vi "Auto_calibrate.vi"(3 "Mode":T4, 5 "Traverse line":T5 {"Row Duration (mins)" format="%#.1f"; "Row No" min=0; "Trace Gas Concentration (%)" min=0.0 format="%#.2f"; "Emission Rate (l/min)" format="%#.2f"; "Tunnel Speed" format="%#.2f"; "Start X" format="%#.2f"; "Start Y" format="%#.2f"; "Start Z" format="%#.2f"; "End X" format="%#.2f"; "End Y" format="%#.2f"; "End Z" format="%#.2f"; "Averaging time (min)" min=0.0 format="%#.2f"}) -> (0 "Error Messages":string, 1 "Status":T2, 2 "Traverse Out":T5 {"Row Duration (mins)" format="%#.1f"; "Row No" min=0; "Trace Gas Concentration (%)" min=0.0 format="%#.2f"; "Emission Rate (l/min)" format="%#.2f"; "Tunnel Speed" format="%#.2f"; "Start X" format="%#.2f"; "Start Y" format="%#.2f"; "Start Z" format="%#.2f"; "End X" format="%#.2f"; "End Y" format="%#.2f"; "End Z" format="%#.2f"; "Averaging time (min)" min=0.0 format="%#.2f"})   [LabVIEW 2010]
uses:
  Gen Trav/Traverse_cluster.ctl
  Gen Trav/Spacing.ctl
  Controls/Multi_run_mode.ctl
  Controls/User_Specific_mode.ctl
  Controls/Auto_Calib_Type.ctl
  Gen Trav/Multi_Run_Status.ctl
  Controls/Auto_Calib_Case.ctl
  File/Setup_Filetype.ctl
  Calibration/Calib_mode.ctl
  Controls/Save_Data.ctl
  Controls/Post_Process.ctl
  Controls/Setup.ctl
  Globals/Meas_global.vi
  Globals/Calib_global.vi
  Globals/Trav_pos_global.vi
  Globals/Plug_in_data_global.vi
  Globals/Extra_Commands_Global.vi
  <vilib>/Analysis/NI_AALBase.lvlib
panel:
  out "Minimum St Dev":dbl[](array[numeric])
  out "Time FFID valve moved":dbl
  out "Wait factor":dbl
  out "Establishment time":string
  out "Orig Calib file string":string
  out "Concentrations":dbl[](array[numeric])
  out "FFID St Dev":dbl[][](array[numeric]) format="%.2f"
  in  "Clear Calib History":bool
  out "Coefficients":dbl[][](array[numeric]) format="%.2f"
  out "Currently in Case":T1
  out "Valve position":dbl format="%.2f"
  out "Currently On":i32
  out "Values":dbl[][](array[numeric]) format="%.2f"
  out "FF Indexes":i16[](array[numeric])
  out "Ch No's":i16[](array[numeric])
  out "No of Calib Points":i32
  out "Root Name":string[](array[string])
  out "Original Calib File":path
  out "Calibration varying":T3
  in  "stop":bool
  out "New Calib Filenames":path[](array[path])
  # "Specific Argument Options\n      Tunnel Speed;1;2;3;4\nOR  Traverse Position\nOR   Concentration"
  # "X           Y            Z"
  # "Start"
  # "End"
  # "X           Y            Z"
  # "Start"
  # "End"
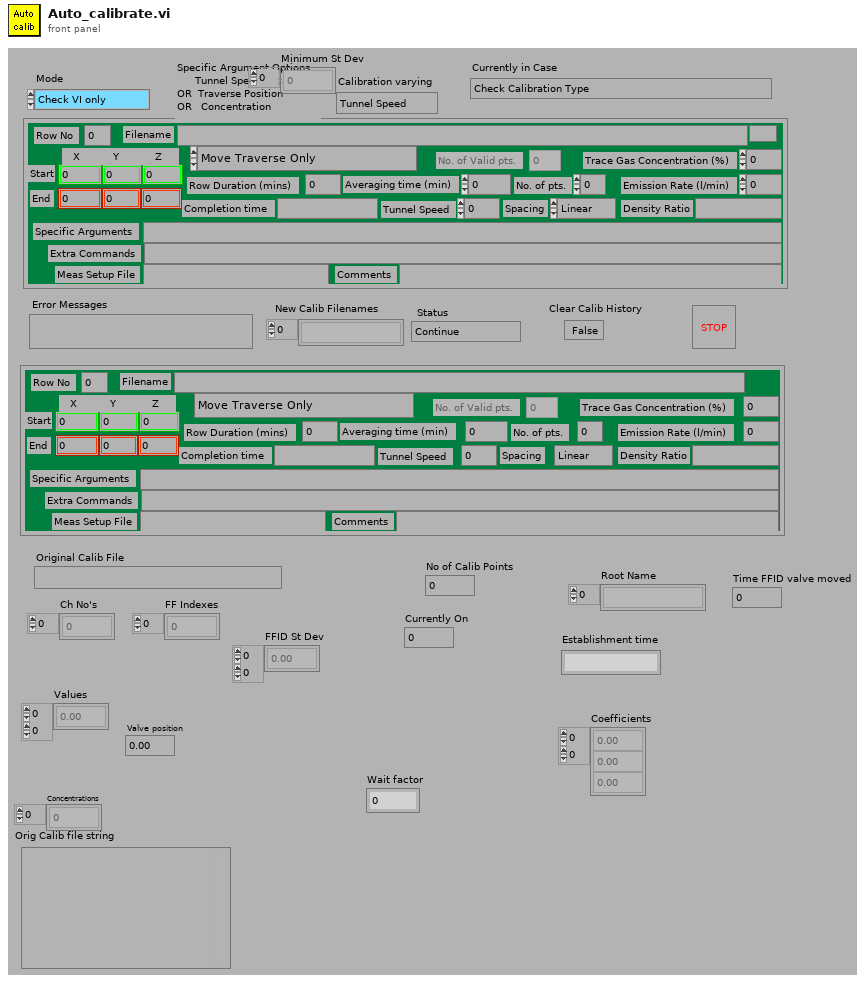
[diagram p1: front panel]
types:
  T1 = typedef "Auto_Calib_Case.ctl" = enum16{"Check Calibration Type", "Check if Original Calib file is Valid", "Get sampling rate etc. from meas setup file", "Setup Calibration Program", "Get Channel Numbers", "Check use latest selected on Mesurement setup files", "Create New Calib Filenames", "Setup Calibration Values in 2D array", "Create Measurement Setup File (Concentration Only)", "Are There Enough Calibration Points", "Set Measurement Conditions", "Measure Calibration Point", "Do Another Calibration Point?", "Skip Next Frame?", "Insert New calibration Filenames into Measurement Setup file", "Warn if FFID calibration is very non linear", "Warn if FFID variance is high", "Insert Bkgnd Variance into calib file", "Warn if FFID voltages are too low", "Warn if Current Calibration fit is poor", "Warn if Calibration Coefficients have significantly altered", "End"}
  T2 = typedef "Multi_Run_Status.ctl" = enum16{"Continue", "Jump to Next Point", "Jump to Next Row", "Jump To Fall Back", "Terminate Run"}
  T3 = typedef "Auto_Calib_Type.ctl" = enum16{"Tunnel Speed", "Traverse Position", "Concentration"}
  T4 = typedef "User_Specific_mode.ctl" = enum16{"Check VI only", "Run VI"}
  T5 = typedef "Traverse_cluster.ctl" = cluster{"Start X":dbl, "Start Y":dbl, "Start Z":dbl, "End X":dbl, "End Y":dbl, "End Z":dbl, "No. of pts.":i32, "Spacing":T6, "Filename":path, "Tunnel Speed":dbl, "Averaging time (min)":dbl, "Extra Commands":string, "Specific Arguments":string, "Emission Rate (l/min)":dbl, "Trace Gas Concentration (%)":dbl, "Density Ratio":string, "Comments":string, "Row No":i32, "Row Type Selector":T7, "Completion time":string, "Row Duration (mins)":dbl, "No. of Valid pts.":i32, "Meas Setup File":string}
  T6 = typedef "Spacing.ctl" = enum16{"Linear", "Log", "Gauss", "Specified", "N/A"}
  T7 = typedef "Multi_run_mode.ctl" = enum16{"Move Traverse Only", "Set Tunnel Speed Only", "Set Source Only", "Set Measurement Conditions", "Single Measurement", "Vertical Profile", "Lateral Profile", "Longitudinal Profile", "Explore Volume", "Multi-Axis Profile", "Auto Calibrate", "Meas Fast FID Bkgnd", "Check Beam Power", "Scanning Valve Measurement", "Run VI Named:", "Set ADAM Ch", "Wait (minutes)", "Send Message", "Synchronize With:", "Fall Back to this Row", "Turn Off Row Repeating", "Blank Row"}
  T8 = typedef "Setup_Filetype.ctl" = enum16{"Measurement Setups", "Calibration Setups", "General", "Results File Plotter Setups", "Speed Calib Tweaks"}
  T9 = typedef "Calib_mode.ctl" = enum16{"Show Setup", "Take a New Calibration Point", "Refit Curve", "Setup Front Panel"}
  T10 = typedef "Save_Data.ctl" = enum16{"Save No Data", "Save Data"}
  T11 = typedef "Post_Process.ctl" = enum16{"Take New Data", "Post Process Raw Data File"}
  T12 = typedef "Setup.ctl" = enum16{"Run Program", "Show Setup", "Save Current Setup", "Setup Front Panel"}
  T13 = typedef "Cal_Inst_type.ctl" = enum16{"Propeller anemometer", "Pressure Transducer", "Hot wire", "Cross wire velocity", "Cross wire angle", "Generic Linear", "Generic Polynomial", "Generic BackPoly", "Fast FID", "Thermocouple", "Cold wire", "Pulsed Wire"}
  T14 = typedef "Ref_Inst_type.ctl" = enum16{"Propellor anemometer", "Pressure Transducer", "Raw voltage", "Pitot-static tube", "Preston tube", "Generic Linear", "Generic Polynomial", "Thermocouple", "LDA", "Enter Value", "ADAM Channel"}
  T15 = cluster{"2nd Ref type":T14, "2nd inst present":bool}
  T16 = cluster{"high limit (10V)":sgl, "low limit (-10V)":sgl, "Ch No":i16, "Var name":string}[]
  T17 = cluster{"high limit (10V)":sgl, "low limit (-10V)":sgl, "Ch No":i16, "Var name":string}
  T18 = typedef "Inst_type.ctl" = enum16{"Propeller anemometer", "Raw voltage", "Pressure Transducer", "Pitot-static tube", "Preston tube", "Hot wire", "Cross wire 1", "Cross wire 2", "Generic Linear", "Generic Polynomial", "Generic BackPoly", "Fast FID", "Thermocouple", "Cold wire", "Pulsed Wire", "LDA Vel", "LDA Tran time", "LDA Arr time"}
  T19 = cluster{"high limit (10V)":sgl, "low limit (-10V)":sgl, "Ch No":i16, "Calib filename":path, "Inst type":T18, "Symbol":string, "Move channel":bool, "Use Latest":bool, "D":dbl, "Ch Name":string}[]
  T20 = typedef "Status_Cluster.ctl" = cluster{"Status":T2, "Error Type":string, "Error Description":string}
  T21 = typedef "Valco_valve_ph.ctl" = u16
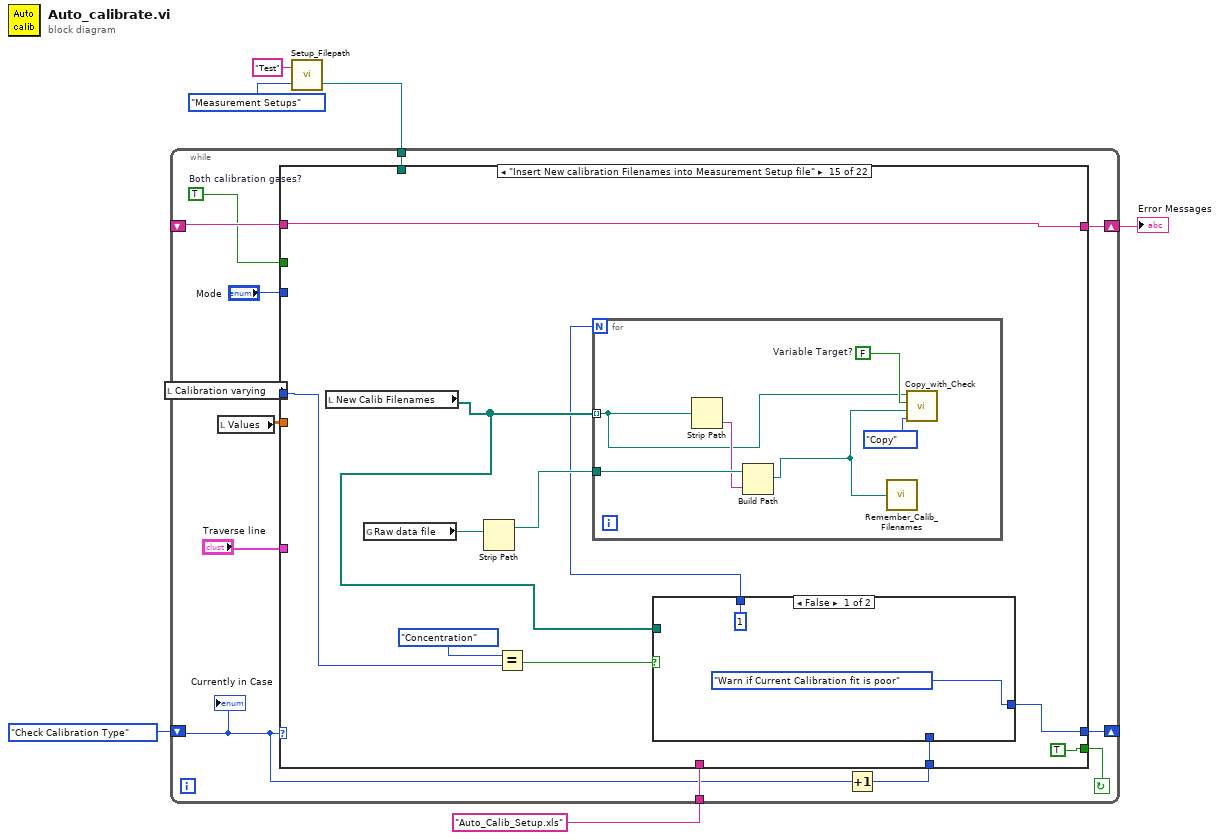
[diagram p0: block diagram]
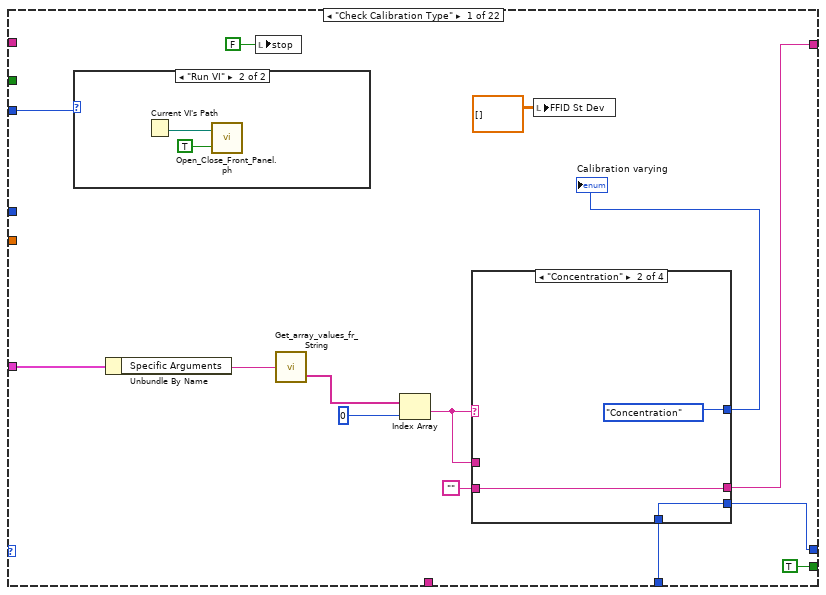
[diagram p2: hidden frame]
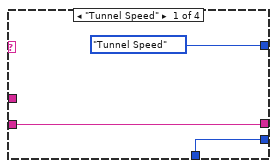
[diagram p4: hidden frame]
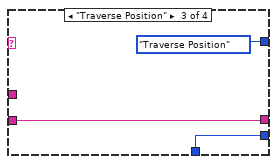
[diagram p5: hidden frame]
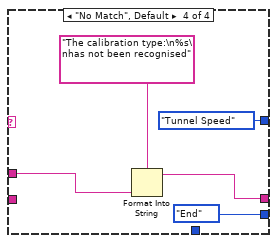
[diagram p6: hidden frame]
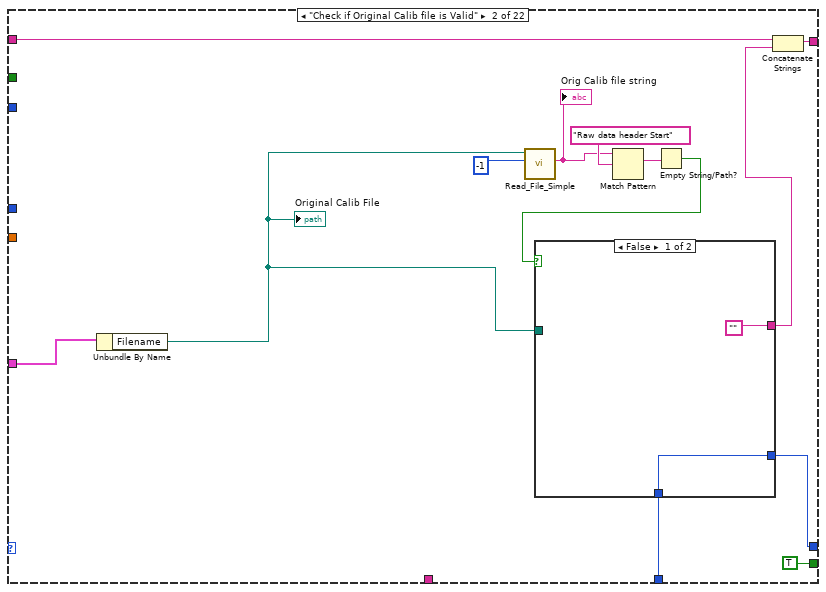
[diagram p7: hidden frame]
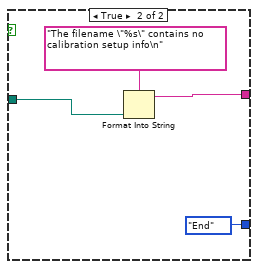
[diagram p8: hidden frame]
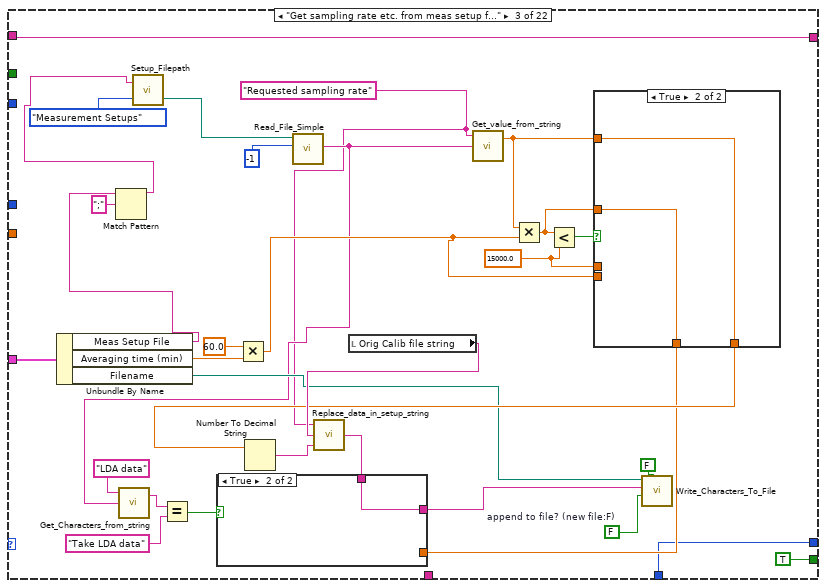
[diagram p9: hidden frame]
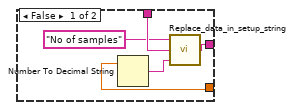
[diagram p10: hidden frame]
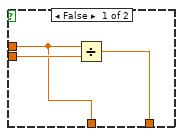
[diagram p11: hidden frame]
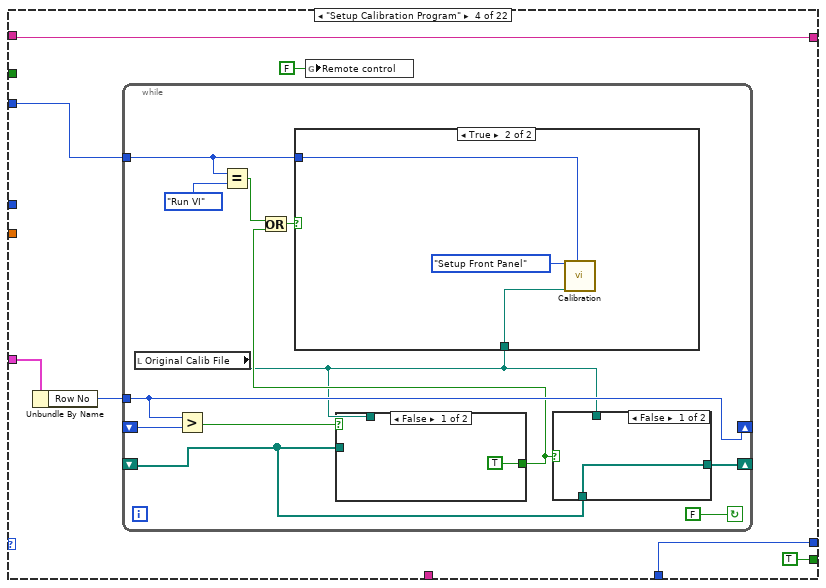
[diagram p12: hidden frame]
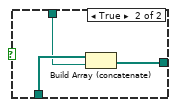
[diagram p13: hidden frame]
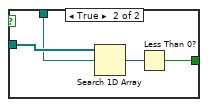
[diagram p15: hidden frame]
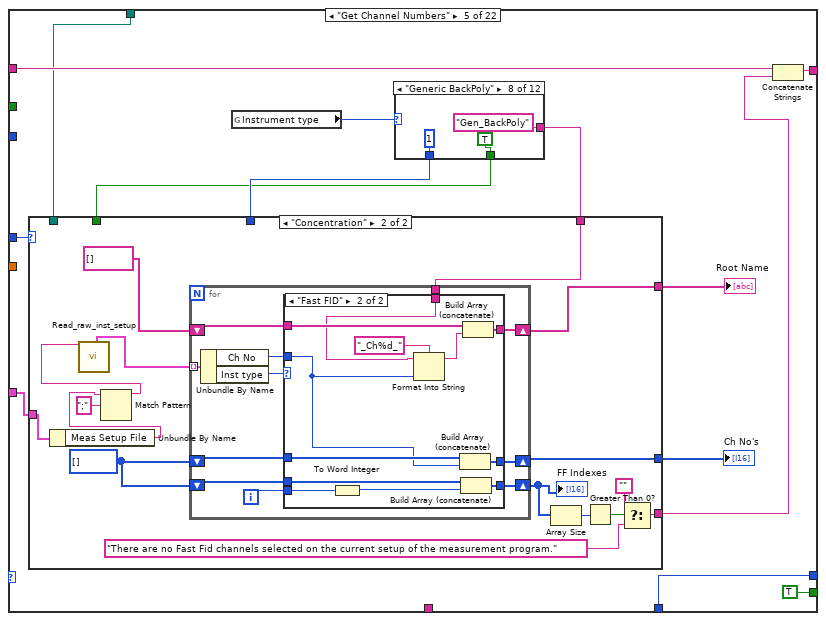
[diagram p16: hidden frame]
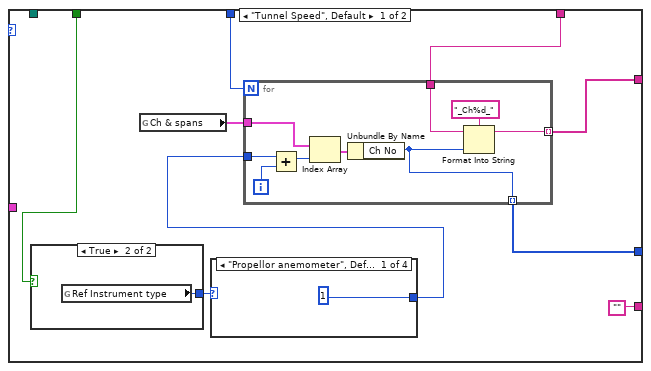
[diagram p17: hidden frame]
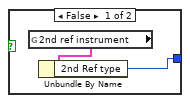
[diagram p18: hidden frame]
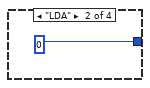
[diagram p19: hidden frame]
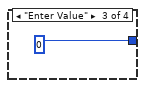
[diagram p20: hidden frame]
diagram:
  n1 = call "Setup_Filepath.vi"("Setup File Type"=Setup_Filetype."Measurement Setups", "Filename in"="Test") -> ("Filename Out"=w2:path)  [unwired: 1 out]
  n2 = while {
    shift-left: _ -> [w11]
    shift-right: [w12] -> w5
    shift-left: Auto_Calib_Case."Check Calibration Type" ("Currently in Case") -> [w10]
    shift-right: [w9] -> _
    tunnel: "Auto_Calib_Setup.xls" -> [w19]
    tunnel: w2 -> [w7]
    stop <- w15 continue-if-true
    w8 = TRUE  # Both calibration gases?
    n3 = local read "Calibration varying"() -> (w14:T3)
    n4 = local read "Values"() -> (w13:dbl[][])
    n5 = Increment(x=w10) -> (x+1=w16:T1)
    n6 = case shown="\"Insert New calibration Filenames into Measurement Setup file\"" w10 {
      tunnel: "Traverse line" -> [w33 w62 w100 w114 w145 _ _ w367 w400 _ w577 _ _ _ _ _ _ _ _ _ w991 w1022]
      tunnel: "Mode" -> [w24 _ _ w115 _ _ w318 _ w401 _ w572 _ w737 _ _ _ _ _ _ _ _ w1023]
      tunnel: w19 -> [_ _ _ _ _ _ _ _ w405 _ _ w649 _ _ _ _ _ _ _ _ _ _]
      tunnel: [w22 w52 w82 w117 w148 w264 w315 w358 w403 w540 w565 w648 w738 w764 w774 w793 w831 w896 w914 w970 w1014 w1028] -> w9
      tunnel: w16 -> [w23 w51 w82 w117 w148 w264 w315 w359 w403 w539 w559 w648 _ w763 w773 w793 w831 w896 w914 w970 w1014 w1028]
      tunnel: [TRUE TRUE TRUE TRUE TRUE TRUE TRUE TRUE w399 TRUE TRUE TRUE TRUE TRUE TRUE TRUE TRUE TRUE TRUE TRUE TRUE FALSE] -> w15
      tunnel: w14 -> [_ _ _ _ w152 _ w314 w365 _ _ w563 w650 w736 w762 w776 _ _ _ _ _ _ w1024]
      tunnel: w13 -> [_ _ _ _ _ _ _ _ w398 w549 w576 _ _ _ _ _ w838 _ w920 _ _ _]
      tunnel: [w26 w54 w80 w118 w149 w265 w329 w362 w404 w543 w560 w646 w735 w767 w780 w802 w845 w892 w921 w959 w1007 w1027] -> w12
      tunnel: w11 -> [_ w56 w80 w118 w151 w265 w329 w361 w404 w544 w560 w646 w735 w767 w780 w802 w845 w892 w921 w959 w1007 w1027]
      tunnel: w8 -> [_ _ _ _ _ _ _ w360 _ _ _ _ _ _ _ _ _ _ _ _ _ w1021]
      tunnel: w7 -> [_ _ _ _ w144 w267 _ _ w402 _ _ _ _ _ _ _ _ _ _ _ _ _]
      frame "Check Calibration Type" {
        n7 = case shown="\"Run VI\"" w24 {
          frame "Check VI only" {
          }
          frame "Run VI" {
            n8 = Current VI's Path() -> (path=w34:path)
            n9 = call "Open_Close_Front_Panel.ph.vi"("Front Panel Window:Open"=TRUE, "VI path"=w34) -> ()  [unwired: 2 out]
          }
        }
        n10 = Unbundle By Name(w33) -> ("Specific Arguments"=w32:string)
        n11 = local write "stop"(FALSE) -> ()
        n12 = call "Get_array_values_fr_String.vi"("String Value"=w32) -> ("String array"=w31:string[])  [unwired: 1 out]
        n13 = Index Array(array=w31, index=0 ("Index")) -> (element=w29:string)
        n14 = case shown="\"Concentration\"" w29 {
          tunnel: [Auto_Calib_Type."Tunnel Speed" ("Calibration varying") Auto_Calib_Type."Concentration" ("Calibration varying") Auto_Calib_Type."Traverse Position" ("Calibration varying") Auto_Calib_Type."Tunnel Speed" ("Calibration varying")] -> w27
          tunnel: w29 -> [_ _ _ w48]
          tunnel: [w37 w40 w43 w46] -> w26
          tunnel: "" -> [w37 w40 w43 _]
          tunnel: w23 -> [w36 w39 w42 _]
          tunnel: [w36 w39 w42 Auto_Calib_Case."End" ("Currently in Case")] -> w22
          frame "Tunnel Speed" {
          }
          frame "Concentration" {
            (unwired) ""
          }
          frame "Traverse Position" {
          }
          frame "No Match", Default {
            n15 = Format Into String(format string="The calibration type:\n%s\nhas not been recognised" ("Format String"), w48) -> (resulting string=w46:string)  [unwired: 2 in, 1 out]
          }
        }
        "Calibration varying" <- w27
        n16 = local write "FFID St Dev"(dbl[][] [] ("FFID Variance")) -> ()
      }
      frame "Check if Original Calib file is Valid" {
        n17 = Unbundle By Name(w62) -> ("Filename"=w50:path)
        "Original Calib File" <- w50
        n18 = call "Read_File_Simple.vi"("Filename"=w50, "number of characters (all:-1)"=-1) -> ("string"=w59:string)  [unwired: 1 in, 7 out]
        "Orig Calib file string" <- w59
        n19 = Match Pattern(string=w59, regular expression="Raw data header Start") -> (match substring=w58:string)  [unwired: 4 out]
        n20 = Empty String/Path?(string/path=w58) -> (empty?=w57:bool)
        n21 = case shown="False" w57 {
          tunnel: w50 -> [_ w68]
          tunnel: ["" w66] -> w55
          tunnel: [w63 Auto_Calib_Case."End" ("Currently in Case")] -> w52
          tunnel: w51 -> [w63 _]
          frame False {
          }
          frame True {
            n22 = Format Into String(format string="The filename \"%s\" contains no calibration setup info\n" ("Format String"), w68) -> (resulting string=w66:string)  [unwired: 2 in, 1 out]
          }
        }
        n23 = Concatenate Strings(w56, w55) -> (w54:string)
      }
      frame "Get sampling rate etc. from meas setup file" {
        w83 = FALSE  # append to file? (new file:F)
        w72 = "Requested sampling rate"
        w90 = 15000.0 ("y")
        n24 = Unbundle By Name(w100) -> ("Meas Setup File"=w78:string, "Averaging time (min)"=w98:dbl, "Filename"=w85:path)
        n25 = Match Pattern(string=w78, regular expression=";") -> (before substring=w70:string)  [unwired: 4 out]
        n26 = call "Setup_Filepath.vi"("Setup File Type"=Setup_Filetype."Measurement Setups", "Filename in"=w70) -> ("Filename Out"=w69:path)  [unwired: 1 out]
        n27 = Multiply(x=60.0, y=w98) -> (x*y=w89:dbl)
        n28 = call "Read_File_Simple.vi"("Filename"=w69, "number of characters (all:-1)"=-1) -> ("string"=w77:string)  [unwired: 1 in, 7 out]
        n29 = call "Get_Characters_from_string.vi"("Input string"=w77, "Variable name"="LDA data") -> ("Value"=w75:string)  [unwired: 1 in, 1 out]
        n30 = Equal?(x=w75, y="Take LDA data") -> (x = y?=w73:bool)
        n31 = local read "Orig Calib file string"() -> (w94:string)
        n32 = call "Get_value_from_string.vi"("Input string"=w77, "Variable name"=w72) -> ("Value"=w93:dbl)  [unwired: 1 in, 1 out]
        n33 = Multiply(x=w93, y=w89) -> (x*y=w88:dbl)
        n34 = Less?(x=w88, y=w90) -> (x < y?=w96:bool)
        n35 = case shown="True" w96 {
          tunnel: w93 -> [_ w111]
          tunnel: [w108 w111] -> w92
          tunnel: w90 -> [w107 _]
          tunnel: w89 -> [w109 _]
          tunnel: [w107 w110] -> w86
          tunnel: w88 -> [_ w110]
          frame False {
            n36 = Divide(x=w107, y=w109) -> (x/y=w108:dbl)
          }
          frame True {
          }
        }
        n37 = Number To Decimal String(number=w92) -> (decimal integer string=w91:string)  [unwired: 1 out]
        n38 = call "Replace_data_in_setup_string.vi"("New data string"=w91, "Input string"=w94, "Variable name"=w72) -> ("Appended string"=w87:string)
        n39 = case shown="True" w73 {
          tunnel: w87 -> [w105 w106]
          tunnel: w86 -> [w102 _]
          tunnel: [w101 w106] -> w84
          frame False {
            n40 = Number To Decimal String(number=w102) -> (decimal integer string=w103:string)  [unwired: 1 out]
            n41 = call "Replace_data_in_setup_string.vi"("New data string"=w103, "Input string"=w105, "Variable name"="No of samples") -> ("Appended string"=w101:string)
          }
          frame True {
          }
        }
        n42 = call "Write_Characters_To_File.vi"("file path (dialog if empty)"=w85, "advisory dialog? (display:T)"=FALSE, "character string"=w84, "append to file? (new file:F)"=w83) -> ()  [unwired: 1 in, 4 out]
      }
      frame "Setup Calibration Program" {
        n43 = Unbundle By Name(w114) -> ("Row No"=w113:i32)
        n44 = while {
          shift-left: _ -> [w122]
          shift-right: [w120] -> _
          tunnel: w113 -> [w129]
          shift-left: _ -> [w130]
          shift-right: [w129] -> _
          tunnel: w115 -> [w127]
          stop <- FALSE continue-if-true
          n45 = local read "Original Calib File"() -> (w121:path)
          n46 = Greater?(x=w129, y=w130) -> (0:w128:bool)
          n47 = Equal?(x=w127, y=User_Specific_mode."Run VI" ("Mode")) -> (x = y?=w125:bool)
          n48 = case shown="False" w128 {
            tunnel: w122 -> [_ w142]
            tunnel: w121 -> [_ w141]
            tunnel: [TRUE w139] -> w123
            frame False {
            }
            frame True {
              n49 = Search 1D Array(1D array=w142, element=w141) -> (index of element=w140:i32)  [unwired: 1 out]
              n50 = Less Than 0?(x=w140) -> (x < 0?=w139:bool)
            }
          }
          n51 = Or(x=w125, y=w123) -> (x .or. y?=w124:bool)
          n52 = case shown="True" w124 {
            tunnel: w127 -> [_ w137]
            tunnel: w121 -> [_ w136]
            frame False {
            }
            frame True {
              n53 = call "Calibration.vi"("Mode"=Calib_mode."Setup Front Panel", "Calib file"=w136, "Simulate/Run"=w137) -> ()  [unwired: 17 out]
            }
          }
          n54 = case shown="False" w123 {
            tunnel: w122 -> [w131 w134]
            tunnel: w121 -> [_ w133]
            tunnel: [w131 w132] -> w120
            frame False {
            }
            frame True {
              n55 = Build Array (concatenate)(w134, w133) -> (w132:path[])
            }
          }
        }
        n56 = global write "Meas_global.vi" "Remote control"(FALSE ("Remote control")) -> ()
      }
      frame "Get Channel Numbers" {
        n57 = global read "Calib_global.vi" "Instrument type"() -> (w156:T13)
        n58 = case shown="\"Generic BackPoly\"" w156 {
          tunnel: ["Prop" "Mano" "HW" "XW" "XW" "Gen_Lin" "Gen_Poly" "Gen_BackPoly" "FF" "Therm" "CW" "PWA"] -> w155
          tunnel: [1 1 1 2 2 1 1 1 1 1 1 1] -> w146
          tunnel: [TRUE TRUE TRUE TRUE FALSE TRUE TRUE TRUE TRUE TRUE TRUE TRUE] -> w143
          frame "Propeller anemometer" {
          }
          frame "Pressure Transducer" {
          }
          frame "Hot wire" {
          }
          frame "Cross wire velocity" {
          }
          frame "Cross wire angle" {
          }
          frame "Generic Linear" {
          }
          frame "Generic Polynomial" {
          }
          frame "Generic BackPoly" {
          }
          frame "Fast FID" {
          }
          frame "Thermocouple" {
          }
          frame "Cold wire" {
          }
          frame "Pulsed Wire" {
          }
        }
        n59 = case shown="\"Concentration\"" w152 {
          tunnel: w155 -> [w163 w197]
          tunnel: [w159 w196] -> w154
          tunnel: [w160 w194] -> w153
          tunnel: ["" w187] -> w150
          tunnel: w146 -> [w161 _]
          tunnel: w145 -> [_ w186]
          tunnel: w144 -> [_ _]
          tunnel: w143 -> [w157 _]
          frame "Tunnel Speed", Default {
            n60 = case shown="True" w157 {
              tunnel: [w166 w168] -> w165
              frame False {
                n61 = global read "Calib_global.vi" "2nd ref instrument"() -> (w167:T15)
                n62 = Unbundle By Name(w167) -> ("2nd Ref type"=w166:T14)
              }
              frame True {
                n63 = global read "Calib_global.vi" "Ref Instrument type"() -> (w168:T14)
              }
            }
            n64 = global read "Calib_global.vi" "Ch & spans"() -> (w162:T16)
            n65 = case shown="\"Propellor anemometer\", Default" w165 {
              tunnel: [1 i16 0 0 0] -> w158
              frame "Propellor anemometer", Default {
              }
              frame "LDA" {
              }
              frame "Enter Value" {
              }
              frame "ADAM Channel" {
              }
            }
            n66 = for {
              N: w161 -> [_]
              tunnel: [w175] -> w160 mode=indexing
              tunnel: w163 -> [w174]
              tunnel: w162 -> [w173]
              tunnel: [w172] -> w159 mode=indexing
              tunnel: w158 -> [w170]
              i -> [w171]
              n67 = Add(x=w170, y=w171) -> (x+y=w169:i32)
              n68 = Index Array(array=w173, index=w169) -> (element=w177:T17)
              n69 = Unbundle By Name(w177) -> ("Ch No"=w175:i16)
              n70 = Format Into String(format string="_Ch%d_" ("Format String"), initial string=w174, w175) -> (resulting string=w172:string)  [unwired: 1 in, 1 out]
            }
          }
          frame "Concentration" {
            w193 = i16[] []
            n71 = Unbundle By Name(w186) -> ("Meas Setup File"=w183:string)
            n72 = Match Pattern(string=w183, regular expression=";") -> (before substring=w182:string)  [unwired: 4 out]
            n73 = call "Read_raw_inst_setup.vi"("Setup file"=w182) -> ("Ch & spans choices"=w185:T19)  [unwired: 18 out]
            n74 = for {
              tunnel: w185 -> [w208] mode=indexing
              tunnel: w197 -> [w207]
              shift-right: [w203] -> w196
              shift-left: string[] [] -> [w204]
              shift-right: [w201] -> w194
              shift-left: w193 -> [w202]
              shift-right: [w200] -> w192
              shift-left: w193 -> [w199]
              i -> [w198]
              n75 = Unbundle By Name(w208) -> ("Ch No"=w206:i16, "Inst type"=w205:T18)
              n76 = case shown="\"Fast FID\"" w205 {
                tunnel: w207 -> [_ w213]
                tunnel: w206 -> [_ w215]
                tunnel: w204 -> [w211 w223]
                tunnel: [w211 w222] -> w203
                tunnel: w202 -> [w210 w221]
                tunnel: [w210 w220] -> w201
                tunnel: w199 -> [w209 w218]
                tunnel: [w209 w219] -> w200
                tunnel: w198 -> [_ w217]
                frame "Generic Linear", Default {
                }
                frame "Fast FID" {
                  n77 = To Word Integer(number=w217) -> (16bit integer=w216:i16)
                  n78 = Format Into String(format string="_Ch%d_", initial string=w213, w215) -> (resulting string=w212:string)  [unwired: 1 in, 1 out]
                  n79 = Build Array (concatenate)(w221, w215) -> (w220:i16[])
                  n80 = Build Array (concatenate)(w218, w216) -> (w219:i16[])
                  n81 = Build Array (concatenate)(w223, w212) -> (w222:string[])
                }
              }
            }
            "FF Indexes" <- w192
            n82 = Array Size(array=w192) -> (size(s)=w191:i32)
            n83 = Greater Than 0?(x=w191) -> (x > 0?=w190:bool)
            n84 = Select(t="", s=w190, f="There are no Fast Fid channels selected on the current setup of the measurement program.") -> (s? t:f=w187:string)
          }
        }
        "Root Name" <- w154
        "Ch No's" <- w153
        n85 = Concatenate Strings(w151, w150) -> (w149:string)
      }
      frame "Check use latest selected on Mesurement setup files" {
        n86 = global read "Trav_pos_global.vi" "Measurement setup files"() -> (w260:string[])
        n87 = local read "Ch No's"() -> (w266:i16[])
        n88 = Build Array (concatenate)(w260, "Current_Setup.xls") -> (w261:string[])
        n89 = for {
          tunnel: w267 -> [w270]
          tunnel: w261 -> [w269] mode=indexing
          tunnel: w266 -> [w268]
          n90 = stacked-sequence {
            seq-local: [w271 _ _] -> [_ w277 w305]
            seq-local: [_ w275 _] -> [_ _ w303]
            tunnel: w270 -> [w274 _ w302]
            tunnel: w269 -> [w273 _ w301]
            tunnel: w268 -> [_ w276 _]
            frame #0 {
              n91 = Build Path(base path=w274, name or relative path=w273) -> (appended path=w272:path)
              n92 = call "Read_File_Simple.vi"("Filename"=w272) -> ("string"=w271:string)  [unwired: 2 in, 7 out]
            }
            frame #1 {
              n93 = while {
                shift-right: [w282] -> w275
                shift-left: w277 -> [w283]
                tunnel: w276 -> [w286]
                i -> [w290]
                stop <- w279 continue-if-true
                n94 = Increment(x=w290) -> (x+1=w284:i32)
                n95 = Format Into String(format string="An ch %d Ch No", w284) -> (resulting string=w289:string)  [unwired: 2 in, 1 out]
                n96 = call "Get_value_from_string.vi"("Input string"=w283, "Variable name"=w289) -> ("Status"=w288:enum16{"Char in string", "Char not in string"}, "Value"=w287:dbl)  [unwired: 1 in]
                n97 = To Long Integer(number=w287) -> (32bit integer=w285:i32)
                n98 = Search 1D Array(1D array=w286, element=w285) -> (index of element=w281:i32)  [unwired: 1 in]
                n99 = Greater Or Equal To 0?(x=w281) -> (x >= 0?=w280:bool)
                n100 = case shown="\"Char in string\"" w288 {
                  tunnel: [TRUE FALSE] -> w279
                  frame "Char in string" {
                  }
                  frame "Char not in string" {
                  }
                }
                n101 = And(x=w280, y=w279) -> (x .and. y?=w278:bool)
                n102 = case shown="True" w278 {
                  tunnel: w284 -> [w294 _]
                  tunnel: w283 -> [w293 w298]
                  tunnel: [w292 w298] -> w282
                  frame True {
                    n103 = Format Into String(format string="An ch %d Use latest Calib", w294) -> (resulting string=w296:string)  [unwired: 2 in, 1 out]
                    n104 = call "Replace_data_in_setup_string.vi"("New data string"="TRUE" ("Replace with"), "Input string"=w293, "Variable name"=w296) -> ("Appended string"=w292:string)
                  }
                  frame False {
                  }
                }
              }
            }
            frame #2 {
              n105 = Equal?(x=w305, y=w303) -> (x = y?=w304:bool)
              n106 = case shown="True" w304 {
                tunnel: w302 -> [w308 _]
                tunnel: w303 -> [w311 _]
                tunnel: w301 -> [w307 _]
                frame False {
                  w310 = FALSE  # append to file? (new file:F)
                  n107 = Build Path(base path=w308, name or relative path=w307) -> (appended path=w306:path)
                  n108 = call "Write_Characters_To_File.vi"("file path (dialog if empty)"=w306, "advisory dialog? (display:T)"=FALSE, "character string"=w311, "append to file? (new file:F)"=w310) -> ()  [unwired: 1 in, 4 out]
                }
                frame True {
                }
              }
            }
          }
        }
      }
      frame "Create New Calib Filenames" {
        n109 = local read "Original Calib File"() -> (w327:path)
        n110 = Get Date/Time String(date format (0)=enum16{"short", "long", "abbreviated"}."short") -> (date string=w322:string)  [unwired: 3 out]
        n111 = Strip Path(path=w327) -> (stripped path=w317:path)  [unwired: 1 out]
        n112 = local read "Root Name"() -> (w313:string[])
        n113 = case shown="\"Tunnel Speed\", Default" w314 {
          tunnel: w313 -> [_ w334]
          tunnel: [1 w333] -> w312
          frame "Tunnel Speed", Default {
          }
          frame "Concentration" {
            n114 = Array Size(array=w334) -> (size(s)=w333:i32)
          }
        }
        n115 = call "Replace_Character.vi"("Replace with"="-", "Input String"=w322, "Search For"="/") -> ("Output string"=w319:string)  [unwired: 1 out]
        n116 = List Folder(path=w317) -> (filenames=w331:string[])  [unwired: 1 in, 5 out]
        n117 = To Upper Case(1:w331) -> (0:w330:string[])
        n118 = for {
          N: w312 -> [_]
          tunnel: w313 -> [w337] mode=indexing
          tunnel: w330 -> [w341]
          tunnel: w317 -> [w340]
          tunnel: [w336] -> w326 mode=indexing
          tunnel: w319 -> [w338]
          tunnel: w318 -> [w335]
          n119 = while {
            tunnel: w337 -> [w348]
            tunnel: w338 -> [w349]
            tunnel: [w344] -> w339
            tunnel: w341 -> [w351]
            i -> [w353]
            stop <- w355 continue-if-true
            n120 = Increment(x=w353) -> (x+1=w350:i32)
            n121 = Format Into String(format string="%s_%d.xls" ("Format String"), initial string=w348, w349, w350) -> (resulting string=w345:string)  [unwired: 1 in, 1 out]
            n122 = call "Replace_Character.vi"("Replace with"="_", "Input String"=w345, "Search For"=" ") -> ("Output string"=w344:string)  [unwired: 1 out]
            n123 = To Upper Case(1:w344) -> (0:w354:string)
            n124 = Search 1D Array(1D array=w351, element=w354) -> (index of element=w356:i32)  [unwired: 1 out]
            n125 = Not Equal?(x=w356, y=-1) -> (x != y?=w355:bool)
          }
          n126 = Build Path(base path=w340, name or relative path=w339) -> (appended path=w336:path)
          n127 = case shown="\"Run VI\"" w335 {
            tunnel: w336 -> [_ w342]
            frame "Check VI only" {
            }
            frame "Run VI" {
              n128 = call "Calibration.vi"("Mode"=Calib_mode."Setup Front Panel", "Calib file"=w342) -> ()  [unwired: 1 in, 17 out]
            }
          }
        }
        "New Calib Filenames" <- w326
        n129 = Index Array(array=w326, index=0 ("Index")) -> (element=w324:path)
        n130 = global write "Meas_global.vi" "Results file"(w324) -> ()
        "Establishment time" <- "!Establish Exp Conditions (s) = 15" ("Message")
      }
      frame "Setup Calibration Values in 2D array" {
        n131 = case shown="\"Concentration\"" w365 {
          tunnel: [w376 w382 w397] -> w364
          tunnel: w367 -> [w371 _ w396]
          tunnel: ["" "" w395] -> w363
          tunnel: w360 -> [_ w380 _]
          tunnel: w359 -> [w370 w379 w394]
          tunnel: [w369 w379 w393] -> w358
          frame "Tunnel Speed" {
            n132 = Unbundle By Name(w371) -> ("Specific Arguments"=w374:string)
            n133 = call "Get_array_values_fr_String.vi"("String Value"=w374) -> ("Numeric Array"=w372:dbl[])  [unwired: 1 out]
            n134 = Array Subset(array=w372, index=1 ("Array Index")) -> (w368:dbl[])  [unwired: 1 in]
            n135 = for {
              tunnel: w368 -> [w378] mode=indexing
              tunnel: [w377] -> w376 mode=indexing
              n136 = Build Array(w378) -> (w377:dbl[])
            }
            n137 = Increment(x=w370) -> (x+1=w369:T1)
          }
          frame "Concentration" {
            n138 = case shown="True" w380 {
              tunnel: [w384 w388] -> w383
              frame True {
                n139 = Build Array(3.0, 2.0, 1.0) -> (w384:dbl[])
              }
              frame False {
                n140 = Build Array(1.0, 3.0) -> (w388:dbl[])
              }
            }
            n141 = for {
              tunnel: w383 -> [w392] mode=indexing
              tunnel: [w391] -> w382 mode=indexing
              n142 = Build Array(w392) -> (w391:dbl[])
            }
          }
          frame "Traverse Position" {
            n143 = call "Create_Pos_array.vi"("Traverse line"=w396) -> ("Error Messages"=w395:string, "Array of Positions"=w397:dbl[][])  [unwired: 5 in, 2 out]
            n144 = Increment(x=w394) -> (x+1=w393:T1)
          }
        }
        "Values" <- w364
        n145 = Concatenate Strings(w361, w363) -> (w362:string)
      }
      frame "Create Measurement Setup File (Concentration Only)" {
        n146 = stacked-sequence {
          seq-local: [w416 _ _ _ _ _ _] -> [_ w435 _ _ _ _ _]
          seq-local: [_ w433 _ _ _ _ _] -> [_ _ w456 _ _ _ _]
          seq-local: [_ _ _ _ w478 _ _] -> [_ _ _ _ _ w491 _]
          seq-local: [_ _ _ _ w483 _ _] -> [_ _ _ _ _ w492 _]
          tunnel: w402 -> [w407 _ w457 _ _ _ _]
          tunnel: w405 -> [_ _ w458 _ _ _ _]
          tunnel: w401 -> [_ _ _ w464 _ w494 w524]
          tunnel: w400 -> [w413 _ _ _ w490 w495 _]
          tunnel: [_ _ _ _ _ w493 _] -> w399
          tunnel: w398 -> [_ _ _ w467 _ _ _]
          frame #0 {
            w420 = TRUE  # Show Dialog?
            n147 = Unbundle By Name(w413) -> ("Meas Setup File"=w414:string)
            n148 = Match Pattern(string=w414, regular expression=";") -> (before substring=w412:string)  [unwired: 4 out]
            n149 = Build Path(base path=w407, name or relative path=w412) -> (appended path=w421:path)
            n150 = Format Into String(format string="Meas Setup File   %s", w407) -> (resulting string=w406:string)  [unwired: 2 in, 1 out]
            n151 = call "Read_spec_No_of_Characters.vi"("Filename"=w421) -> ("character string"=w422:string)  [unwired: 1 out]
            n152 = call "Get_string_subset.vi"("String Name"=w406, "Show Dialog?"=w420, "String to split"=w422, "File Label"="Raw data header") -> ("Output string"=w409:string)  [unwired: 1 out]
            n153 = call "Get_value_from_string.vi"("Input string"=w409, "Variable name"="No of analogue inst") -> ("Value"=w410:dbl)  [unwired: 1 in, 1 out]
            n154 = for {
              N: w410 -> [_]
              shift-right: [w424] -> w419
              shift-left: w409 -> [w426]
              i -> [w430]
              n155 = Increment(x=w430) -> (x+1=w429:i32)
              n156 = Number To Decimal String(number=w429) -> (decimal integer string=w432:string)  [unwired: 1 out]
              n157 = Concatenate Strings("An ch ", w432, " Inst type") -> (w427:string)
              n158 = call "Replace_data_in_setup_string.vi"("New data string"="Raw voltage", "Input string"=w426, "Variable name"=w427) -> ("Appended string"=w424:string)
            }
            n159 = call "Replace_data_in_setup_string.vi"("New data string"="No LDA data", "Input string"=w419, "Variable name"="LDA data" ("Label for characters")) -> ("Appended string"=w416:string)
          }
          frame #1 {
            n160 = global read "Calib_global.vi" "New Setup String"() -> (w436:string)
            n161 = for {
              N: 4 -> [_]
              shift-right: [w441] -> w433
              shift-left: w435 -> [w442]
              tunnel: w436 -> [w438]
              i -> [w440]
              n162 = case shown="3" w440 {
                tunnel: [w445 w448 w451 "No of blocks"] -> w439
                tunnel: w438 -> [w444 w447 w450 _]
                tunnel: [w443 w446 w449 "1" ("Value")] -> w437
                frame 0, Default {
                  w445 = "No of samples"
                  n163 = call "Get_Characters_from_string.vi"("Input string"=w444, "Variable name"=w445) -> ("Value"=w443:string)  [unwired: 1 in, 1 out]
                }
                frame 2 {
                  w448 = "Actual sampling rate"
                  n164 = call "Get_Characters_from_string.vi"("Input string"=w447, "Variable name"=w448) -> ("Value"=w446:string)  [unwired: 1 in, 1 out]
                }
                frame 3 {
                  w451 = "Board type"
                  n165 = call "Get_Characters_from_string.vi"("Input string"=w450, "Variable name"=w451) -> ("Value"=w449:string)  [unwired: 1 in, 1 out]
                }
                frame 1 {
                }
              }
              n166 = call "Replace_data_in_setup_string.vi"("New data string"=w437, "Input string"=w442, "Variable name"=w439) -> ("Appended string"=w441:string)
            }
          }
          frame #2 {
            w462 = FALSE  # advisory dialog? (display:T)
            w463 = FALSE  # append to file? (new file:F)
            n167 = call "Remove_Plug_Ins_etc.vi"("Input String"=w456) -> ("Output string"=w455:string)
            n168 = call "Add_label_to_string.vi"("String to write"=w455, "File Label"="Raw data header") -> ("Output string"=w459:string)
            n169 = Build Path(base path=w457, name or relative path=w458) -> (appended path=w454:path)
            n170 = call "Add_length_to_string.vi"("String in"=w459) -> ("String out"=w461:string)
            n171 = call "Write_Characters_To_File.vi"("file path (dialog if empty)"=w454, "advisory dialog? (display:T)"=w462, "character string"=w461, "append to file? (new file:F)"=w463) -> ()  [unwired: 1 in, 4 out]
          }
          frame #3 {
            w466 = 0 ("Index")
            w471 = 0.0 ("Input Element")
            n172 = Index Array(array=w467, index (row)=w466, index (col)=w466) -> (element=w465:dbl)
            n173 = case shown="\"Run VI\"" w464 {
              tunnel: w465 -> [_ w474]
              frame "Check VI only" {
              }
              frame "Run VI" {
                n174 = flat-sequence {
                  tunnel: w474 -> [w475]
                  frame #0 {
                    n175 = call "Fast_FID_Valve_Control.vi"("Requested Position"=w475) -> ()  [unwired: 7 out]
                  }
                  frame #1 {
                    n176 = Get Date/Time In Seconds() -> (seconds since 1Jan1904=w477:timestamp)
                    n177 = To Double Precision Float(number=w477) -> (double precision float=→"Time FFID valve moved":dbl)
                  }
                }
              }
            }
            n178 = Build Array("GMU:Calibration:Gas 1", "GMU:Calibration:Gas 2") -> (w473:string[])
            n179 = call "Get_Current_Scan_client.vi"("ADAM Ch Names"=w473) -> ("Numerical Values"=w472:dbl[])  [unwired: 3 out]
            n180 = Build Array (concatenate)(w471, w471, w472, w471) -> (→"Concentrations":dbl[])
          }
          frame #4 {
            n181 = Unbundle By Name(w490) -> ("Extra Commands"=w489:string, "Start X"=w487:dbl, "Start Y"=w486:dbl, "Start Z"=w485:dbl)
            n182 = Build Array(w487, w486, w485) -> (w483:dbl[])
            n183 = call "Which_Trav_Setup.vi"("Extra Command String"=w489) -> ("Traverse Setup"=w488:string)
            n184 = call "Read_Traverse_Pos_File.vi"("Traverse Name"=w488) -> ("Tunnel Coordinates"=w484:dbl[])
            n185 = Subtract(x=w484, y=w483) -> (x-y=w482:dbl[])
            n186 = Absolute Value(x=w482) -> (abs(x)=w481:dbl[])
            n187 = Less?(x=w481, y=0.5) -> (x < y?=w479:bool[])
            n188 = And Array Elements(Boolean array=w479) -> (logical AND=w478:bool)
          }
          frame #5 {
            n189 = case shown="False" w491 {
              tunnel: w495 -> [w505 _]
              tunnel: w494 -> [w501 _]
              tunnel: [w497 TRUE] -> w493
              tunnel: w492 -> [w496 _]
              frame False {
                w500 = dbl[] [30.0, 15.0, 0.0] ("appended array")
                n190 = call "Coordinate_Trans_.vi"("Input Position"=w496) -> ("X"=w502:dbl, "Y"=w503:dbl, "Z"=w504:dbl)
                n191 = Array Size(array=w500) -> (size(s)=w499:i32)
                n192 = Decrement(x=w499) -> (x-1=w498:i32)
                n193 = while {
                  tunnel: w501 -> [w514]
                  tunnel: w505 -> [w520]
                  tunnel: w500 -> [w519] mode=indexing
                  tunnel: w504 -> [w517]
                  tunnel: w503 -> [w516]
                  tunnel: w502 -> [w515]
                  tunnel: w498 -> [w510]
                  tunnel: [w506] -> w497
                  i -> [w511]
                  stop <- w507 continue-if-true
                  n194 = Add(x=w517, y=w519) -> (x+y=w518:dbl)
                  n195 = Less?(x=w511, y=w510) -> (x < y?=w508:bool)
                  n196 = Bundle By Name(cluster=w520, "Start X"=w515, "Start Y"=w516, "Start Z"=w518) -> (w521:T5)
                  n197 = call "Set_Traverse_Position.vi"("Simulate/Run"=w514, "Currently on Point"=1, "Traverse line"=w521) -> ("Status Cluster"=w509:T20)  [unwired: 2 out]
                  n198 = Unbundle By Name(w509) -> ("Status"=w512:T2)
                  n199 = call "Prog_Status_Handler.vi"("Status Cluster"=w509, "Simulate/Run"=w514) -> ()  [unwired: 2 out]
                  n200 = local write "Status"(w512) -> ()
                  n201 = Equal?(x=w512, y=Multi_Run_Status."Continue" ("Status")) -> (x = y?=w506:bool)
                  n202 = And(x=w506, y=w508) -> (x .and. y?=w507:bool)
                }
              }
              frame True {
              }
            }
          }
          frame #6 {
            n203 = case shown="\"Run VI\"" w524 {
              frame "Check VI only", Default {
              }
              frame "Run VI" {
                n204 = while {
                  shift-right: [w536] -> _
                  shift-left: _ -> [w537]
                  tunnel: [w535] -> w530
                  stop <- TRUE stop-if-true
                  n205 = Get Date/Time In Seconds() -> (seconds since 1Jan1904=w536:timestamp)
                  n206 = Subtract(x=w536, y=w537) -> (x-y=w535:dbl)
                }
                n207 = Divide(x=w530, y=3600.0) -> (x/y=w529:dbl)
                n208 = Multiply(x=w529, y=0.2) -> (x*y=w527:dbl)
                n209 = Add(x=w527, y=0.8) -> (x+y=w525:dbl)
                n210 = In Range and Coerce(upper limit=2.0, x=w525, lower limit=1.0) -> (coerced(x)=→"Wait factor":dbl)  [unwired: 1 out]
              }
            }
          }
        }
      }
      frame "Are There Enough Calibration Points" {
        n211 = Array Size(array=w549) -> (size(s)=w550:i32[])
        n212 = Index Array(array=w550, index=0 ("Index")) -> (element=w545:i32)
        "No of Calib Points" <- w545
        n213 = Greater?(x=w545, y=1) -> (0:w546:bool)
        n214 = case shown="False" w546 {
          tunnel: ["Less than two calibration points have been specified\n" ""] -> w542
          tunnel: [Auto_Calib_Case."End" ("Currently in Case") w554] -> w540
          tunnel: w539 -> [_ w554]
          frame False {
          }
          frame True {
          }
        }
        n215 = Concatenate Strings(w544, w542) -> (w543:string)
        "Currently On" <- 1 ("Currently On")
      }
      frame "Set Measurement Conditions" {
        n216 = local read "Currently On"() -> (w564:i32)
        n217 = Decrement(x=w564) -> (x-1=w575:i32)
        n218 = Index Array(array=w576, index (row)=w575) -> (element=w574:dbl[])  [unwired: 1 in]
        n219 = case shown="\"Concentration\"" w563 {
          tunnel: w574 -> [w592 w609 w626]
          tunnel: w572 -> [_ _ w624]
          tunnel: w577 -> [w590 w605 w615]
          tunnel: [w591 w604 w613] -> w558
          tunnel: w564 -> [w586 _ w616]
          tunnel: [w589 w603 w620] -> w556
          frame "Tunnel Speed" {
            n220 = Index Array(array=w592, index=0 ("Index")) -> (element=w579:dbl)
            n221 = while {
              shift-right: [w600] -> w581
              shift-left: _ -> [w599]
              tunnel: w579 -> [w602]
              tunnel: [w600] -> w588
              tunnel: [w599] -> w587
              stop <- FALSE continue-if-true
              n222 = Greater Than 0?(x=w602) -> (x > 0?=w600:bool)
            }
            n223 = Exclusive Or(1:w587, 2:w588) -> (0:w584:bool)
            n224 = Greater?(x=w586, y=1) -> (0:w583:bool)
            n225 = And(x=w584, y=w583) -> (x .and. y?=w582:bool)
            n226 = case shown="False" w581 {
              tunnel: [w594 w596] -> w580
              tunnel: w579 -> [w595 w596]
              frame False {
                n227 = Negate(x=w595) -> (-x=w594:dbl)
              }
              frame True {
              }
            }
            n228 = case shown="True" w582 {
              frame False {
              }
              frame True {
                n229 = call "Wait_Seconds_with_display.vi"("Message"="Please rotate the probe you are calibrating", "Seconds to wait"=10000.0) -> ()  [unwired: 2 out]
              }
            }
            n230 = local read "Establishment time"() -> (w589:string)
            n231 = Bundle By Name(cluster=w590, "Tunnel Speed"=w580) -> (w591:T5)
          }
          frame "Traverse Position" {
            n232 = Index Array(array=w609, index=0 ("Index")) -> (element=w608:dbl)
            n233 = Index Array(array=w609, index=1 ("Index")) -> (element=w607:dbl)
            n234 = Index Array(array=w609, index=2 ("Index")) -> (element=w606:dbl)
            n235 = local read "Establishment time"() -> (w603:string)
            n236 = Bundle By Name(cluster=w605, "Start X"=w608, "Start Y"=w607, "Start Z"=w606) -> (w604:T5)
          }
          frame "Concentration" {
            w614 = nan ("Start X")
            n237 = local read "Wait factor"() -> (w619:dbl)
            n238 = Index Array(array=w626, index=0 ("Index")) -> (element=w617:dbl)
            n239 = case shown="3" w616 {
              tunnel: [w628 w636 100.0] -> w618
              tunnel: w619 -> [w634 w637 _]
              frame 1, Default {
                n240 = local read "Time FFID valve moved"() -> (w631:dbl)
                n241 = Get Date/Time In Seconds() -> (seconds since 1Jan1904=w633:timestamp)
                n242 = Multiply(x=w634, y=35.0) -> (x*y=w630:dbl)
                n243 = To Double Precision Float(number=w633) -> (double precision float=w632:dbl)
                n244 = Subtract(x=w632, y=w631) -> (x-y=w629:dbl)
                n245 = Subtract(x=w630, y=w629) -> (x-y=w628:dbl)
              }
              frame 2 {
                n246 = Multiply(x=w637, y=25.0) -> (x*y=w636:dbl)
              }
              frame 3 {
              }
            }
            n247 = case shown="\"Run VI\"" w624 {
              tunnel: w617 -> [w641 w642]
              tunnel: [w640 w643] -> w625
              frame "Check VI only" {
                n248 = To Long Integer(number=w641) -> (32bit integer=w640:i32)
              }
              frame "Run VI" {
                n249 = call "Fast_FID_Valve_Control.vi"("Requested Position"=w642) -> ("Achieved Posn."=w643:T21)  [unwired: 6 out]
              }
            }
            n250 = Number To Decimal String(number=w618) -> (decimal integer string=w621:string)  [unwired: 1 out]
            n251 = Concatenate Strings("!Establish Exp Conditions (s) = " ("Message"), w621) -> (w620:string)
            n252 = To Double Precision Float(number=w625) -> (double precision float=→"Valve position":dbl)
            n253 = Bundle By Name(cluster=w615, "Start X"=w614, "Start Y"=w614, "Start Z"=w614) -> (w613:T5)
          }
        }
        n254 = call "Add_Extra_Command.vi"("Traverse line"=w558, "Extra Command"=w556) -> ("Traverse line Out"=w557:T5)
        n255 = call "Set_Measurement_Conditions.vi"("Simulate/Run"=w572, "Currently on Point"=1, "Traverse line"=w557) -> ("Status Cluster"=w562:T20)  [unwired: 2 out]
        n256 = Unbundle By Name(w562) -> ("Status"=w561:T2)
        "Status" <- w561
        n257 = Equal?(x=w561, y=Multi_Run_Status."Continue" ("Status")) -> (x = y?=w568:bool)
        n258 = Equal?(x=User_Specific_mode."Run VI" ("Mode"), y=w572) -> (x = y?=w569:bool)
        n259 = Increment(x=w559) -> (x+1=w566:T1)
        n260 = And(x=w568, y=w569) -> (x .and. y?=w567:bool)
        n261 = Select(t=w559, s=w567, f=w566) -> (s? t:f=w565:T1)
      }
      frame "Measure Calibration Point" {
        n262 = case shown="\"Concentration\"" w650 {
          tunnel: w649 -> [_ w659]
          tunnel: [w653 w658] -> w645
          tunnel: [w651 w657] -> w644
          frame "Tunnel Speed", Default {
            n263 = local read "New Calib Filenames"() -> (w654:path[])
            n264 = Index Array(array=w654, index=0 ("Index")) -> (element=w655:path)
            n265 = call "Calibration.vi"("Mode"=Calib_mode."Take a New Calibration Point", "Calib file"=w655) -> ("Coefficients"=w651:dbl[][], "Status Out"=w653:T2)  [unwired: 1 in, 15 out]
          }
          frame "Concentration" {
            # "St Dev"
            # "Mean"
            n266 = stacked-sequence {
              seq-local: [_ w663 _] -> [_ _ w707]
              seq-local: [_ w662 _] -> [_ _ w706]
              tunnel: w659 -> [_ w666 _]
              tunnel: [_ w664 _] -> w658
              tunnel: [_ _ w708] -> w657
              frame #0 {
                n267 = global write "Meas_global.vi" "Remote control"(TRUE ("Remote control")) -> ()
                n268 = global write "Meas_global.vi" "Raw data option"(enum16{"Save raw data", "Raw data not saved"}."Save raw data" ("Raw data option")) -> ()
              }
              frame #1 {
                n269 = local read "New Calib Filenames"() -> (w667:path[])
                n270 = Index Array(array=w667, index=0 ("Index")) -> (element=w665:path)
                n271 = while {
                  tunnel: [w675] -> w664
                  tunnel: w665 -> [w674]
                  tunnel: w666 -> [w672]
                  tunnel: [w671] -> w663
                  tunnel: [w670] -> w662
                  i -> [w669]
                  stop <- w673 continue-if-true
                  n272 = stacked-sequence {
                    seq-local: [_ w677 _ _] -> [_ _ _ w700]
                    seq-local: [_ _ w685 _] -> [_ _ _ w704]
                    tunnel: [_ w677 _ _] -> w675
                    tunnel: w674 -> [_ w682 _ _]
                    tunnel: [_ _ _ w695] -> w673
                    tunnel: w672 -> [_ w678 _ _]
                    tunnel: [_ _ w686 _] -> w671
                    tunnel: [_ _ w685 _] -> w670
                    tunnel: w669 -> [_ _ _ w702]
                    frame #0 {
                      n273 = global write "Meas_global.vi" "Remote control"(TRUE ("Remote control")) -> ()
                    }
                    frame #1 {
                      n274 = call "Get_Data_Base_file_code.vi"("Results Filename"=w682, "Data Type"="Raw_Calibrations") -> ("Raw Data File Name"=w679:path)  [unwired: 3 out]
                      n275 = call "Measurement.vi"("setup"=Setup."Run Program", "Post Process"=Post_Process."Take New Data", "File"=Save_Data."Save No Data", "Raw data file"=w679, "Setup filename"=w678) -> ("Status Out"=w677:T2)  [unwired: 2 in, 12 out]
                    }
                    frame #2 {
                      n276 = local read "FF Indexes"() -> (w688:i16[])
                      n277 = global read "Plug_in_data_global.vi" "Equi Spaced"() -> (w687:dbl[][])
                      n278 = for {
                        tunnel: w688 -> [w694] mode=indexing
                        tunnel: [w692] -> w686 mode=indexing
                        tunnel: [w691] -> w685 mode=indexing
                        tunnel: w687 -> [w693]
                        n279 = Index Array(array=w693, index (row)=w694) -> (element=w690:dbl[])  [unwired: 1 in]
                        n280 = call "De-spiked_Stats.vi"("Raw Signal"=w690, "No of st dev to chop at"=6.0) -> ("mean"=w692:dbl, "standard deviation"=w691:dbl)  [unwired: 1 out]
                      }
                    }
                    frame #3 {
                      n281 = Greater?(x=w704, y=0.15) -> (0:w703:bool[])
                      n282 = Or Array Elements(Boolean array=w703) -> (logical OR=w697:bool)
                      n283 = Less?(x=w702, y=2) -> (x < y?=w698:bool)
                      n284 = Equal?(x=w700, y=Multi_Run_Status."Continue" ("Status Out")) -> (x = y?=w696:bool)
                      n285 = Compound Arithmetic op=AND(w696, w697, w698) -> (w695:bool)
                    }
                  }
                }
              }
              frame #2 {
                n286 = local read "FFID St Dev"() -> (w711:dbl[][])
                n287 = local read "Valve position"() -> (w715:dbl)
                n288 = local read "Concentrations"() -> (w709:dbl[])
                n289 = global read "Meas_global.vi" "Temp"() -> (w716:dbl)
                n290 = Build Array (concatenate)(w707, w706) -> (w710:dbl[])
                n291 = Build Array (concatenate)(w711, w710) -> (→"FFID St Dev":dbl[][])
                n292 = Index Array(array=w709, index=w715) -> (element=w714:dbl)
                n293 = local read "New Calib Filenames"() -> (w713:path[])
                n294 = for {
                  tunnel: w707 -> [w722] mode=indexing
                  tunnel: w716 -> [w721]
                  tunnel: w714 -> [w720]
                  tunnel: [w719] -> w708 mode=indexing
                  tunnel: w713 -> [w718] mode=indexing
                  tunnel: w706 -> [w717] mode=indexing
                  n295 = stacked-sequence {
                    tunnel: w722 -> [w728 _]
                    tunnel: w721 -> [w725 _]
                    tunnel: w720 -> [w727 _]
                    tunnel: [_ w730] -> w719
                    tunnel: w718 -> [_ w729]
                    tunnel: w717 -> [w723 _]
                    frame #0 {
                      n296 = Build Array(w727, w728, w723, 0.0 ("element"), w725) -> (w726:dbl[])
                      n297 = global write "Calib_global.vi" "Calibration Points"(w726) -> ()
                    }
                    frame #1 {
                      n298 = call "Calibration.vi"("Mode"=Calib_mode."Refit Curve", "Calib file"=w729) -> ("Coefficients"=w731:dbl[][])  [unwired: 1 in, 16 out]
                      n299 = Index Array(array=w731, index (row)=0 ("Index")) -> (element=w730:dbl[])  [unwired: 1 in]
                    }
                  }
                }
              }
            }
          }
        }
        "Coefficients" <- w644
        n300 = local write "Status"(w645) -> ()
      }
      frame "Do Another Calibration Point?" {
        n301 = local read "No of Calib Points"() -> (w747:i32)
        n302 = local read "Status"() -> (w743:T2)
        n303 = local read "Currently On"() -> (w739:i32)
        n304 = case shown="\"Terminate Run\"" w743 {
          tunnel: [w757 w758 TRUE w761] -> w745
          tunnel: [w757 w758 FALSE w761] -> w746
          frame "Continue", Default {
            w757 = TRUE
          }
          frame "Jump to Next Point" {
            w758 = TRUE
          }
          frame "Jump to Next Row" {
          }
          frame "Terminate Run" {
            w761 = FALSE
          }
        }
        n305 = Greater?(x=w747, y=w739) -> (0:w744:bool)
        n306 = Compound Arithmetic op=AND(invert "stop", w745) -> (w742:bool)
        n307 = Compound Arithmetic op=AND(w742, w746, w744) -> (w740:bool)
        n308 = case shown="False" w740 {
          tunnel: w739 -> [_ w756]
          tunnel: [w750 Auto_Calib_Case."Set Measurement Conditions" ("Currently in Case")] -> w738
          tunnel: w737 -> [w751 _]
          tunnel: w736 -> [w749 _]
          frame False {
            n309 = case shown="\"Check VI only\"" w751 {
              tunnel: [Auto_Calib_Case."End" ("Currently in Case") Auto_Calib_Case."Skip Next Frame?" ("Currently in Case")] -> w750
              tunnel: w749 -> [_ _]
              frame "Check VI only" {
              }
              frame "Run VI" {
              }
            }
          }
          frame True {
            n310 = Increment(x=w756) -> (x+1=w755:i32)
            n311 = local write "Currently On"(w755) -> ()
          }
        }
        n312 = case shown="True" "stop" {
          frame False {
          }
          frame True {
            n313 = local write "Status"(Multi_Run_Status."Terminate Run" ("Status")) -> ()
          }
        }
      }
      frame "Skip Next Frame?" {
        n314 = local read "Status"() -> (w765:T2)
        n315 = case shown="\"Tunnel Speed\", Default" w762 {
          frame "Tunnel Speed", Default {
          }
          frame "Concentration" {
            n316 = call "Fast_FID_Valve_Control.vi"("Requested Position"=4 ("Requested Posn.")) -> ()  [unwired: 7 out]
          }
        }
        n317 = case shown="\"Continue\"" w765 {
          tunnel: [w769 Auto_Calib_Case."End" ("Currently in Case")] -> w764
          tunnel: w763 -> [w769 _]
          frame "Continue" {
          }
          frame "Terminate Run", Default {
          }
        }
      }
      frame "Insert New calibration Filenames into Measurement Setup file" {
        n318 = local read "New Calib Filenames"() -> (w772:path[])
        n319 = global read "Meas_global.vi" "Raw data file"() -> (w779:path)
        n320 = Strip Path(path=w779) -> (stripped path=w778:path)  [unwired: 1 out]
        n321 = Equal?(x=Auto_Calib_Type."Concentration" ("Calibration varying"), y=w776) -> (x = y?=w775:bool)
        n322 = case shown="False" w775 {
          tunnel: [Auto_Calib_Case."Warn if Current Calibration fit is poor" ("Currently in Case") w786] -> w774
          tunnel: w773 -> [_ w786]
          tunnel: w772 -> [_ w785]
          tunnel: [1 w784] -> w771
          frame False {
          }
          frame True {
            n323 = Array Size(array=w785) -> (size(s)=w784:i32)
          }
        }
        n324 = for {
          N: w771 -> [_]
          tunnel: w772 -> [w788] mode=indexing
          tunnel: w778 -> [w792]
          w790 = FALSE  # Variable Target?
          n325 = Strip Path(path=w788) -> (name=w791:string)  [unwired: 1 out]
          n326 = Build Path(base path=w792, name or relative path=w791) -> (appended path=w787:path)
          n327 = call "Remember_Calib_Filenames.vi"("Filename to Remember"=w787) -> ()  [unwired: 1 out]
          n328 = call "Copy_with_Check.vi"("Mode"=enum16{"Move", "Copy"}."Copy", "Target Path"=w787, "Variable Target?"=w790, "Source Path"=w788) -> ()  [unwired: 1 out]
        }
      }
      frame "Warn if FFID calibration is very non linear" {
        w809 = FALSE  # Dialog Box (T)
        n329 = local read "Root Name"() -> (w808:string[])
        n330 = local read "Coefficients"() -> (w811:dbl[][])
        n331 = for {
          tunnel: w811 -> [w818] mode=indexing
          shift-right: [w820] -> w806
          shift-left: "" -> [w821]
          tunnel: w808 -> [w822] mode=indexing
          tunnel: [w815] -> w801 mode=indexing
          tunnel: "If the calibration fit for %s had been linear instead of a second order polynomial, it would have yielded an average fit error of %.1f%%.\\n" ("Format String") -> [w813]
          n332 = Index Array(array=w818, index=0 ("Index")) -> (element=w816:dbl)
          n333 = Absolute Value(x=w816) -> (abs(x)=w815:dbl)
          n334 = Less?(x=w815, y=2.2) -> (x < y?=w819:bool)
          n335 = case shown="False" w819 {
            tunnel: w822 -> [w824 _]
            tunnel: w815 -> [w825 _]
            tunnel: w821 -> [w828 w829]
            tunnel: [w826 w829] -> w820
            tunnel: w813 -> [w823 _]
            frame False {
              n336 = Format Into String(format string=w823, w824, w825) -> (resulting string=w827:string)  [unwired: 2 in, 1 out]
              n337 = Concatenate Strings(w828, w827) -> (w826:string)
            }
            frame True {
            }
          }
        }
        n338 = Array Max & Min(array=w801) -> (max value=w800:dbl)  [unwired: 3 out]
        n339 = Greater?(x=w800, y=7.0) -> (0:w798:bool)
        n340 = Select(t="Very Poor FFID Linearity", s=w798, f="Poor FFID Linearity") -> (s? t:f=w795:string)
        n341 = Empty String/Path?(string/path=w806) -> (empty?=w805:bool)
        n342 = Not(x=w805) -> (.not. x?=w804:bool)
        n343 = Bundle By Name(cluster=errorcluster {"status"=FALSE, "code"=0, "source"=""} ("error in (no error)"), "source"=w806, "status"=w804) -> (w803:errorcluster)
        n344 = call "EnFlo_Error_Handler.vi"("error in (no error)"=w803, "Error Type"=w795, "Dialog Box (T)"=w809) -> ()  [unwired: 3 out]
      }
      frame "Warn if FFID variance is high" {
        w851 = FALSE  # Dialog Box (T)
        n345 = local read "New Calib Filenames"() -> (w833:path[])
        n346 = local read "FFID St Dev"() -> (w853:dbl[][])
        n347 = Index Array(array=w838, index (col)=0 ("disabled index (col)")) -> (element=w836:dbl[])  [unwired: 1 in]
        n348 = Array Size(array=w833) -> (size(s)=w832:i32)
        n349 = for {
          tunnel: w853 -> [w870]
          shift-right: [w872] -> w849
          shift-left: "" -> [w873]
          tunnel: w833 -> [w861] mode=indexing
          tunnel: "For %s the measurement at %dppm had a standard deviation of %.2f volts for an average value of  %.1f volts.\\n" ("Format String") -> [w871]
          tunnel: w836 -> [w864]
          tunnel: [w863] -> w834 mode=indexing
          tunnel: w832 -> [w859]
          tunnel: [w855] -> w830 mode=indexing
          i -> [w858]
          n350 = Add(x=w859, y=w858) -> (x+y=w857:i32)
          n351 = Strip Path(path=w861) -> (name=w860:string)  [unwired: 1 out]
          n352 = Index Array(array=w870, index (col)=w858) -> (element=w862:dbl[])  [unwired: 1 in]
          n353 = Index Array(array=w870, index (col)=w857) -> (element=w856:dbl[])  [unwired: 1 in]
          n354 = Array Max & Min(array=w856) -> (min value=w855:dbl)  [unwired: 3 out]
          n355 = call <vilib>:"Mean.vi"("X"=w862) -> ("mean"=w869:dbl)  [unwired: 1 out]
          n356 = Divide(x=w856, y=w869) -> (x/y=w868:dbl[])
          n357 = Array Max & Min(array=w868) -> (max value=w863:dbl, max index (indices)=w865:i32)  [unwired: 2 out]
          n358 = Greater?(x=w863, y=0.06) -> (0:w866:bool)
          n359 = case shown="True" w866 {
            tunnel: w860 -> [_ w884]
            tunnel: w873 -> [w874 w890]
            tunnel: [w874 w888] -> w872
            tunnel: w871 -> [_ w887]
            tunnel: w865 -> [_ w885]
            tunnel: w864 -> [_ w886]
            tunnel: w863 -> [_ _]
            tunnel: w856 -> [_ w883]
            tunnel: w862 -> [_ w881]
            frame False {
            }
            frame True {
              n360 = local read "Concentrations"() -> (w879:dbl[])
              n361 = Index Array(array=w886, index=w885) -> (element=w880:dbl)
              n362 = Index Array(array=w883, index=w885) -> (element=w877:dbl)
              n363 = Index Array(array=w881, index=w885) -> (element=w882:dbl)
              n364 = Index Array(array=w879, index=w880) -> (element=w878:dbl)
              n365 = Multiply(x=w877, y=2.5) -> (x*y=w876:dbl)
              n366 = Format Into String(format string=w887, w884, w878, w876, w882) -> (resulting string=w889:string)  [unwired: 2 in, 1 out]
              n367 = Concatenate Strings(w890, w889) -> (w888:string)
            }
          }
        }
        "Minimum St Dev" <- w830
        n368 = Array Max & Min(array=w834) -> (max value=w844:dbl)  [unwired: 3 out]
        n369 = Greater?(x=w844, y=0.09) -> (0:w842:bool)
        n370 = Select(t="Very unstable FFID calibration point", s=w842, f="Unstable FFID calibration point") -> (s? t:f=w839:string)
        n371 = Empty String/Path?(string/path=w849) -> (empty?=w848:bool)
        n372 = Not(x=w848) -> (.not. x?=w847:bool)
        n373 = Bundle By Name(cluster=errorcluster {"status"=FALSE, "code"=0, "source"=""} ("error in (no error)"), "source"=w849, "status"=w847) -> (w846:errorcluster)
        n374 = call "EnFlo_Error_Handler.vi"("error in (no error)"=w846, "Error Type"=w839, "Dialog Box (T)"=w851) -> ()  [unwired: 3 out]
      }
      frame "Insert Bkgnd Variance into calib file" {
        n375 = local read "New Calib Filenames"() -> (w893:path[])
        n376 = local read "Minimum St Dev"() -> (w894:dbl[])
        n377 = local read "Coefficients"() -> (w891:dbl[][])
        n378 = for {
          tunnel: w894 -> [w899] mode=indexing
          tunnel: w893 -> [w905] mode=indexing
          tunnel: w891 -> [w902] mode=indexing
          n379 = call "Read_File_Simple.vi"("Filename"=w905) -> ("string"=w909:string)  [unwired: 2 in, 7 out]
          n380 = Index Array(array=w902, index=2) -> (element=w900:dbl)
          n381 = Multiply(x=w899, y=w900) -> (x*y=w898:dbl)
          n382 = Square(x=w898) -> (x^2=w897:dbl)
          n383 = Number To Fractional String(number=w897, precision (6)=i16 8) -> (F-format string=w907:string)  [unwired: 2 out]
          n384 = call "Replace_data_in_setup_string.vi"("New data string"=w907, "Input string"=w909, "Variable name"="Fast FID Bkgnd Variance") -> ("Appended string"=w904:string)
          n385 = call "Write_File_Simple.vi"("append to file? (new file:F)"=FALSE, "character string"=w904, "file path"=w905) -> ()  [unwired: 2 out]
        }
      }
      frame "Warn if FFID voltages are too low" {
        w927 = FALSE  # Dialog Box (T)
        n386 = local read "Coefficients"() -> (w917:dbl[][])
        n387 = local read "Concentrations"() -> (w913:dbl[])
        n388 = Index Array(array=w920, index (col)=0 ("disabled index (col)")) -> (element=w912:dbl[])  [unwired: 1 in]
        n389 = local read "New Calib Filenames"() -> (w916:path[])
        n390 = for {
          tunnel: w913 -> [w932]
          tunnel: w912 -> [w931] mode=indexing
          tunnel: [w930] -> w911 mode=indexing
          n391 = Index Array(array=w932, index=w931) -> (element=w930:dbl)
        }
        n392 = Array Max & Min(array=w911) -> (max value=w910:dbl)  [unwired: 3 out]
        n393 = for {
          shift-right: [w942] -> w925
          shift-left: "" -> [w943]
          tunnel: "For %s the maximum measured calibration voltage was %.1f volts.\nCheck that the FID is running and correctly connected to the acquisition system." ("Format String") -> [w941]
          tunnel: w917 -> [w939] mode=indexing
          tunnel: w916 -> [w935] mode=indexing
          tunnel: w910 -> [w934]
          n394 = Split 1D Array(array=w939, index=1) -> (second subarray=w938:dbl[])  [unwired: 1 out]
          n395 = call "Polybackwards.vi"("Coefficients"=w938, "Y input"=w934) -> ("X output"=w933:dbl)  [unwired: 1 out]
          n396 = Less?(x=w933, y=0.2) -> (x < y?=w936:bool)
          n397 = case shown="True" w936 {
            tunnel: w943 -> [w944 w951]
            tunnel: [w944 w949] -> w942
            tunnel: w941 -> [_ w948]
            tunnel: w935 -> [_ w947]
            tunnel: w933 -> [_ w945]
            frame False {
            }
            frame True {
              n398 = Strip Path(path=w947) -> (name=w946:string)  [unwired: 1 out]
              n399 = Format Into String(format string=w948, w946, w945) -> (resulting string=w950:string)  [unwired: 2 in, 1 out]
              n400 = Concatenate Strings(w951, w950) -> (w949:string)
            }
          }
        }
        n401 = Empty String/Path?(string/path=w925) -> (empty?=w924:bool)
        n402 = Not(x=w924) -> (.not. x?=w923:bool)
        n403 = Bundle By Name(cluster=errorcluster {"status"=FALSE, "code"=0, "source"=""} ("error in (no error)"), "source"=w925, "status"=w923) -> (w922:errorcluster)
        n404 = call "EnFlo_Error_Handler.vi"("error in (no error)"=w922, "Error Type"="Low FFID calibration voltages", "Dialog Box (T)"=w927) -> ()  [unwired: 3 out]
      }
      frame "Warn if Current Calibration fit is poor" {
        w966 = FALSE  # Dialog Box (T)
        n405 = local read "Root Name"() -> (w965:string[])
        n406 = local read "Coefficients"() -> (w968:dbl[][])
        n407 = for {
          tunnel: w968 -> [w975] mode=indexing
          shift-right: [w977] -> w963
          shift-left: "" -> [w978]
          tunnel: w965 -> [w979] mode=indexing
          tunnel: [w972] -> w958 mode=indexing
          n408 = Index Array(array=w975, index=0 ("Index")) -> (element=w973:dbl)
          n409 = Absolute Value(x=w973) -> (abs(x)=w972:dbl)
          n410 = Less?(x=w972, y=1.0) -> (x < y?=w976:bool)
          n411 = case shown="True" w976 {
            tunnel: w979 -> [w981 _]
            tunnel: w972 -> [w982 _]
            tunnel: w978 -> [w985 w986]
            tunnel: [w983 w986] -> w977
            frame False {
              n412 = Format Into String(format string="The calibration for %s has an average fit error of %.1f%%\\n" ("Format String"), w981, w982) -> (resulting string=w984:string)  [unwired: 2 in, 1 out]
              n413 = Concatenate Strings(w985, w984) -> (w983:string)
            }
            frame True {
            }
          }
        }
        n414 = Array Max & Min(array=w958) -> (max value=w957:dbl)  [unwired: 3 out]
        n415 = Greater?(x=w957, y=7.0) -> (0:w955:bool)
        n416 = Select(t="Very Poor Calibration", s=w955, f="Poor Calibration") -> (s? t:f=w952:string)
        n417 = Empty String/Path?(string/path=w963) -> (empty?=w962:bool)
        n418 = Not(x=w962) -> (.not. x?=w961:bool)
        n419 = Bundle By Name(cluster=errorcluster {"status"=FALSE, "code"=0, "source"=""} ("error in (no error)"), "source"=w963, "status"=w961) -> (w960:errorcluster)
        n420 = call "EnFlo_Error_Handler.vi"("error in (no error)"=w960, "Error Type"=w952, "Dialog Box (T)"=w966) -> ()  [unwired: 3 out]
      }
      frame "Warn if Calibration Coefficients have significantly altered" {
        w1012 = FALSE  # Dialog Box (T)
        w999 = 8.0 ("y")
        n421 = local read "New Calib Filenames"() -> (w1004:path[])
        n422 = local read "Root Name"() -> (w1003:string[])
        n423 = global read "Calib_global.vi" "Instrument type"() -> (w1002:T13)
        n424 = Unbundle By Name(w991) -> ("Extra Commands"=w990:string)
        n425 = global read "Extra_Commands_Global.vi" "If Command"() -> (w992:string)
        n426 = call "Extra_Commands.vi"("String to Search"=w990, "Command"=w992) -> ("String Value"=w989:string)  [unwired: 1 in, 4 out]
        n427 = call "Calibration_Analysis.vi"("Root Name"=w1003, "New Calib Filenames"=w1004, "Instrument type"=w1002, "Clear Calib History"="Clear Calib History") -> ("Error String"=w1001:string, "Max % Error"=w987:dbl)
        n428 = call "Get_array_values_fr_String.vi"("String Value"=w989) -> ("Numeric Array"=w988:dbl[], "String array"=w994:string[])
        n429 = Greater?(x=w987, y=w999) -> (0:w1000:bool)
        n430 = Index Array(array=w994, index=0 ("Index")) -> (element=w995:string)
        n431 = case shown="\"Drift Greater Than\"" w995 {
          tunnel: w988 -> [w1018 _]
          tunnel: w987 -> [w1017 _]
          frame "Drift Greater Than" {
            n432 = Index Array(array=w1018, index=1 ("Index")) -> (element=w1016:dbl)
            n433 = Greater?(x=w1017, y=w1016) -> (0:w1015:bool)
            n434 = case shown="True" w1015 {
              frame False {
              }
              frame True {
                n435 = local write "Status"(Multi_Run_Status."Jump To Fall Back" ("Status")) -> ()
              }
            }
          }
          frame "No Match", Default {
          }
        }
        n436 = Format Into String(format string="Calibration Drift Greater than %d%%", w999) -> (resulting string=w997:string)  [unwired: 2 in, 1 out]
        n437 = Select(t=w997, s=w1000, f="Calibration Drift") -> (s? t:f=w1005:string)
        n438 = Empty String/Path?(string/path=w1001) -> (empty?=w1010:bool)
        n439 = Not(x=w1010) -> (.not. x?=w1009:bool)
        n440 = Bundle By Name(cluster=errorcluster {"status"=FALSE, "code"=0, "source"=""} ("error in (no error)"), "source"=w1001, "status"=w1009) -> (w1008:errorcluster)
        n441 = call "EnFlo_Error_Handler.vi"("error in (no error)"=w1008, "Error Type"=w1005, "Dialog Box (T)"=w1012) -> ()  [unwired: 3 out]
      }
      frame "End" {
        n442 = local read "Original Calib File"() -> (w1025:path)
        n443 = Bundle By Name(cluster=w1022, "Filename"=w1025) -> ()  [unwired: 1 out]
        n444 = case shown="\"Concentration\"" w1024 {
          tunnel: w1022 -> [_ w1041]
          tunnel: w1023 -> [_ w1029]
          tunnel: w1021 -> [_ w1040]
          frame "Tunnel Speed", Default {
          }
          frame "Concentration" {
            n445 = Unbundle By Name(w1041) -> ("Averaging time (min)"=w1043:dbl)
            n446 = global read "Trav_pos_global.vi" "Simulation Time"() -> (w1032:timestamp)
            n447 = Unbundle By Name(w1041) -> ("Start X"=w1049:dbl, "Start Y"=w1048:dbl, "Start Z"=w1047:dbl)
            n448 = Build Array(w1049, w1048, w1047) -> (w1050:dbl[])
            n449 = Select(t=3 ("No. of pts."), s=w1040, f=2 ("No. of pts.")) -> (s? t:f=w1034:i32)
            n450 = call "Coordinate_Trans_.vi"("Input Position"=w1050) -> ("X"=w1046:dbl, "Y"=w1045:dbl, "Z"=w1044:dbl)
            n451 = Multiply(x=60.0, y=w1043) -> (x*y=w1037:dbl)
            n452 = Add(x=w1044, y=50.0) -> (x+y=w1051:dbl)
            n453 = Add(x=w1037, y=60.0) -> (x+y=w1035:dbl)
            n454 = Bundle By Name(cluster=w1041, "Start X"=w1046, "Start Y"=w1045, "Start Z"=w1051) -> (w1052:T5)
            n455 = Multiply(x=w1035, y=w1034) -> (x*y=w1033:dbl)
            n456 = Add(x=w1032, y=w1033) -> (x+y=w1030:timestamp)
            n457 = call "Set_Traverse_Position.vi"("Simulate/Run"=w1029, "Currently on Point"=1, "Traverse line"=w1052) -> ()  [unwired: 3 out]
            n458 = call "Run_FFID_Bkgnd.vi"("Simulated Time"=w1030, "Run Now?"=TRUE, "Simulate/Run"=w1029) -> ()  [unwired: 3 out]
          }
        }
        "Traverse Out" <- w1022
      }
    }
    "Currently in Case" <- w10
  }
  "Error Messages" <- w5
